vi "qHDT.vi"(0 "System no.":i32=1 min=1 max=4 step=1, 2 "DeviceID to query":i32[](array[numeric]), 3 "DeviceAxis to query":i32[](array[numeric]), 4 "All DeviceIDs?":bool, 5 "error in":errorcluster) -> (15 "TableID":i32[](array[numeric]), 16 "DeviceID to query out":i32[](array[numeric]), 17 "DeviceAxis to query out":i32[](array[numeric]), 19 "error out":errorcluster)   [LabVIEW 2026]
doc: "Returns the lookup table which is currently assigned to the axis of the Human Interface Device (HID). See controller user manual for details.\n\nC-867:"
panel:
  # "Returns the lookup table which is currently assigned to the axis of the Human Interface \nDevice (HID)."
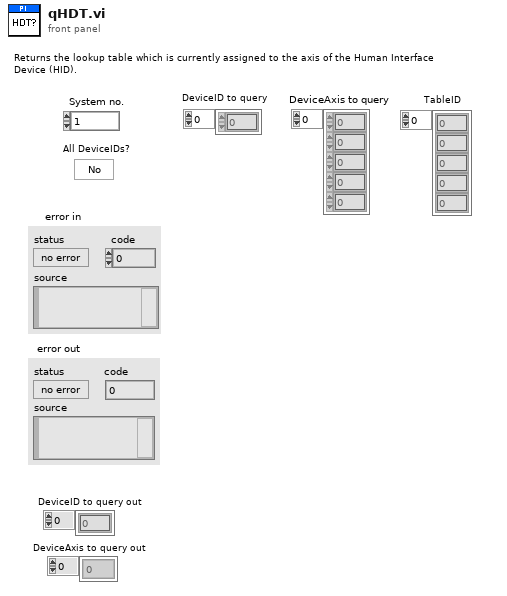
[diagram p1: front panel]
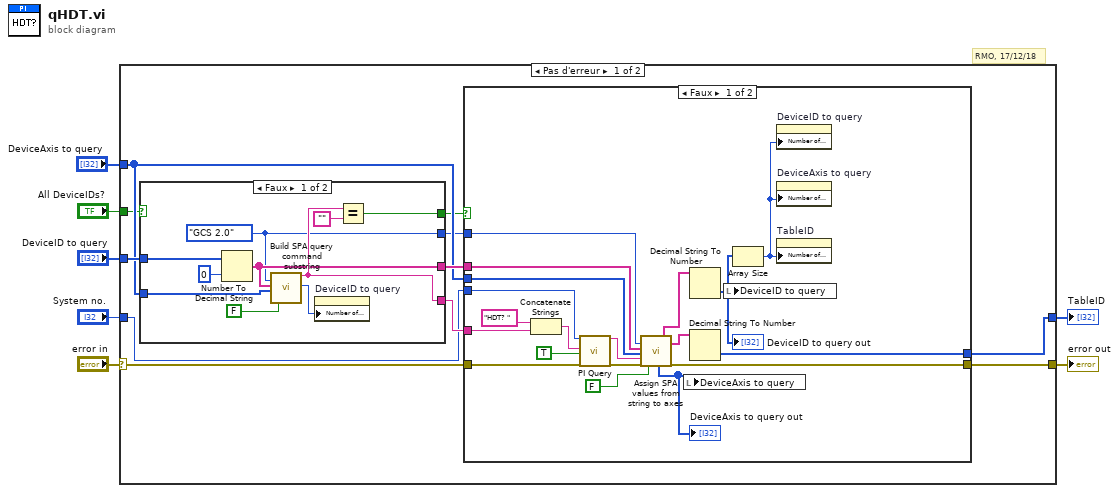
[diagram p0: block diagram]
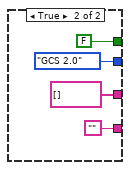
[diagram p2: hidden frame]
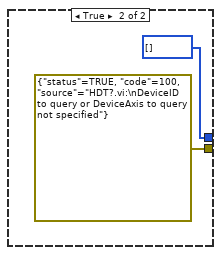
[diagram p3: hidden frame]
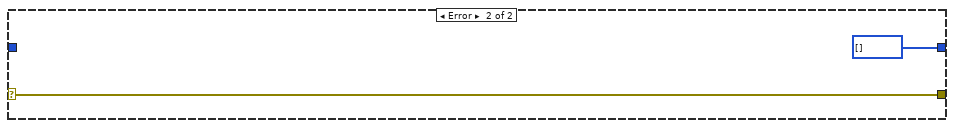
[diagram p4: hidden frame]
diagram:
  # "RMO, 17/12/18"
  n1 = case shown="Pas d'erreur" "error in" {
    selector: "error in" -> [w8 w54]
    tunnel: "DeviceID to query" -> [w18 _]
    tunnel: "System no." -> [w10 _]
    tunnel: "DeviceAxis to query" -> [w15 _]
    tunnel: [w14 w54] -> w4
    tunnel: "All DeviceIDs?" -> [w12 _]
    tunnel: [w11 i32[] []] -> w2
    frame No Error {
      n2 = case shown="Faux" w12 {
        tunnel: w18 -> [w21 _]
        tunnel: [w28 "" ("Command substring")] -> w17
        tunnel: [w20 string[] [] ("Designator to query")] -> w16
        tunnel: w15 -> [w27 _]
        tunnel: [w26 FALSE] -> w13
        tunnel: [w19 enum16{"GCS 1.0", "GCS 2.0"}."GCS 2.0" ("Syntax")] -> w9
        frame False {
          w19 = enum16{"GCS 1.0", "GCS 2.0"}."GCS 2.0" ("Syntax")
          n3 = Number To Decimal String(number=w21, width (-)=i16 0) -> (decimal integer string=w20:string[])
          n4 = call "Build SPA query command substring.vi"("Syntax"=w19, "Axes to query"=w20, "Parameter number"=w27, "Parameter no. format \n(Decimal: FALSE)"=FALSE ("Parameter no. format \n(Decimal: FALSE)")) -> ("Command substring"=w28:string, "Number of rows"=w24:u32)  [unwired: 3 in, 11 out]
          n5 = property on="DeviceID to query" class="Tabl (strict)"("Number of Rows"=w24) -> ()  [unwired: 2 in, 2 out]
          n6 = Equal?(x=w28, y="" ("x")) -> (x = y?=w26:bool)
        }
        frame True {
        }
      }
      n7 = case shown="Faux" w13 {
        tunnel: w8 -> [w45 _]
        tunnel: w17 -> [w48 _]
        tunnel: w16 -> [w47 _]
        tunnel: w10 -> [w44 _]
        tunnel: w15 -> [w46 _]
        tunnel: [w33 errorcluster {"status"=TRUE, "code"=100, "source"="HDT?.vi:\nDeviceID to query or DeviceAxis to query not specified"} ("error out")] -> w14
        tunnel: [w38 i32[] []] -> w11
        tunnel: w9 -> [w43 _]
        frame False {
          n8 = Concatenate Strings("HDT? ", w48) -> (w49:string)
          n9 = call "PI Query.vi"("System no."=w44, "String to send"=w49, "Attach termination char.?"=TRUE ("Attach Linefeed?"), "error in"=w45) -> ("String read"=w34:string, "error out"=w35:errorcluster)  [unwired: 3 in, 11 out]
          n10 = call "Assign SPA values from string to axes.vi"("Syntax"=w43, "Queried axes"=w47, "Parameter no."=w46, "Input string"=w34, "error in"=w35, "Parameter no. format \n(Decimal: FALSE)"=FALSE ("Parameter no. format \n(Decimal: FALSE)")) -> ("Parameter no. out"=w41:i32[], "Queried axes out"=w40:string[], "Parameter strings"=w39:string[], "error out"=w33:errorcluster)  [unwired: 2 in, 8 out]
          "DeviceAxis to query out" <- w41
          n11 = local write "DeviceAxis to query"(w41) -> ()
          n12 = Decimal String To Number(string=w40) -> (number=w37:i32[])  [unwired: 3 out]
          "DeviceID to query out" <- w37
          n13 = Decimal String To Number(string=w39) -> (number=w38:i32[])  [unwired: 3 out]
          n14 = local write "DeviceID to query"(w37) -> ()
          n15 = Array Size(array=w37) -> (size(s)=w36:i32)
          n16 = property on="DeviceID to query" class="Tabl (strict)"("Number of Rows"=w36) -> ()  [unwired: 2 in, 2 out]
          n17 = property on="DeviceAxis to query" class="Tabl (strict)"("Number of Rows"=w36) -> ()  [unwired: 2 in, 2 out]
          n18 = property on="TableID" class="Tabl (strict)"("Number of Rows"=w36) -> ()  [unwired: 2 in, 2 out]
        }
        frame True {
        }
      }
    }
    frame Error {
    }
  }
  "error out" <- w4
  "TableID" <- w2
